vi "VIDoc Settings Editor.vi"(8 "Error in":errorcluster caption="Error in (no error)", 11 "VIDoc Settings Directory":path) -> (0 "Error out":errorcluster)   [LabVIEW 2023]
uses:
  Settings/VIDoc Settings/VIDoc Settings.lvclass
  Settings/Parser Settings/Parser Settings.lvclass
  Settings/Printer Settings/Printer Settings.lvclass
  <vilib>/event_ctls.llb/usereventprio.ctl
  VIDoc Editor/VIDocEditor.lvclass
  C:/Projects/Open Source/DMC VIDoc - Core/Source/Settings/VIDoc Settings/VIDoc Settings.lvclass
  C:/Projects/Open Source/DMC VIDoc - Core/Source/Editors/VIDoc Editor/VIDocEditor.lvclass
  C:/Projects/Open Source/DMC VIDoc - Core/Source/Settings/Parser Settings/Parser Settings.lvclass
  C:/Projects/Open Source/DMC VIDoc - Core/Source/Settings/Printer Settings/Printer Settings.lvclass
panel:
  in  "JSON Settings Path":path
  in  "Save":bool
  in  "Settings Sections":i32(listbox)
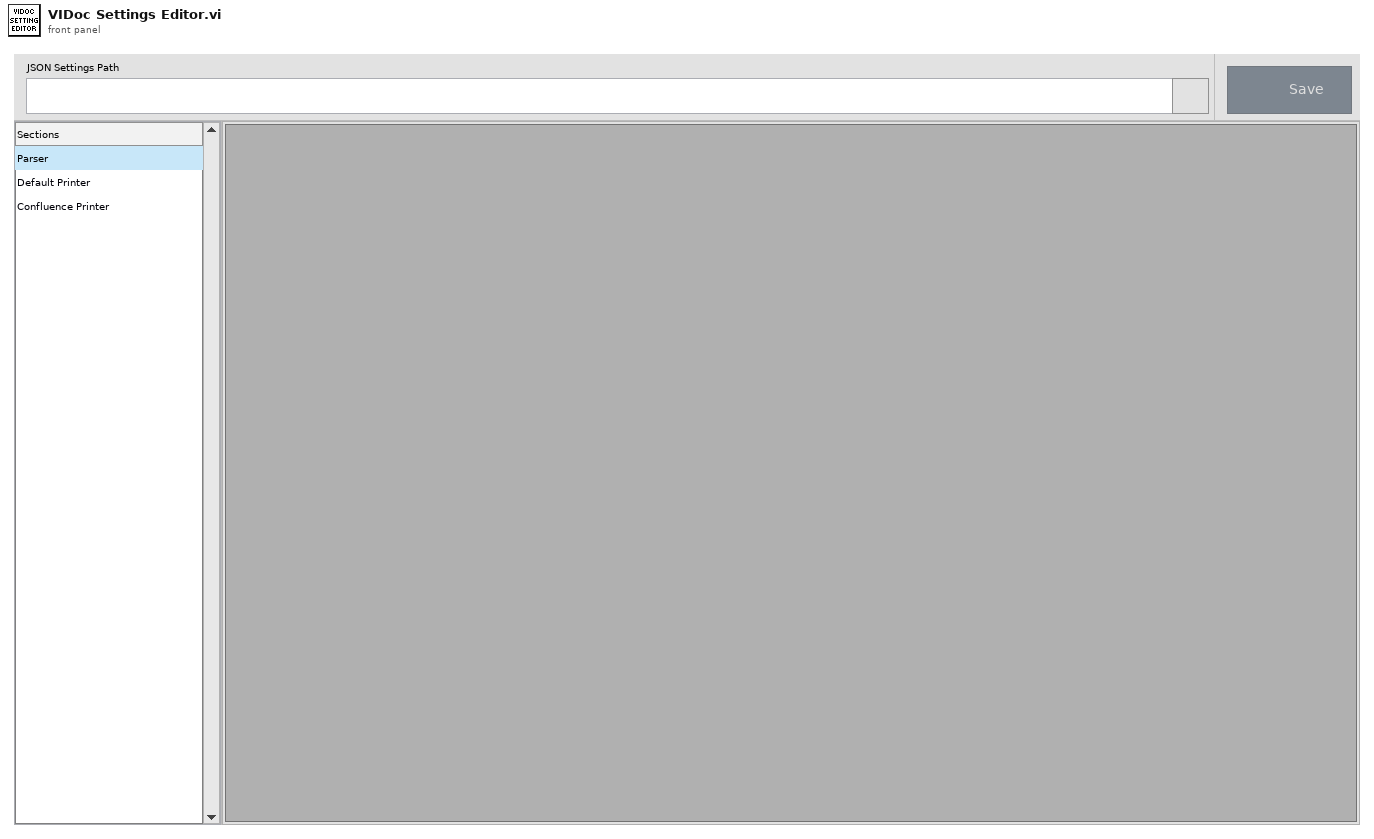
[diagram p1: front panel]
types:
  T1 = enum8{"Enabled", "Disabled", "Disabled and Grayed Out"}
  T2 = cluster{"JSON Settings Path":path, "Editors":refnum<class "VIDoc Settings.lvclass">[], "Current VI":refnum<vi>}
  T3 = typedef "VIDocEditor.lvclass/Editor Events Cluster.ctl" = cluster{"Close":refnum<user-event>, "Revert":refnum<user-event>, "Save":refnum<user-event>, "Changes?":refnum<user-event>}
  T4 = typedef "usereventprio.ctl" = enum32{"high priority", "normal priority"}
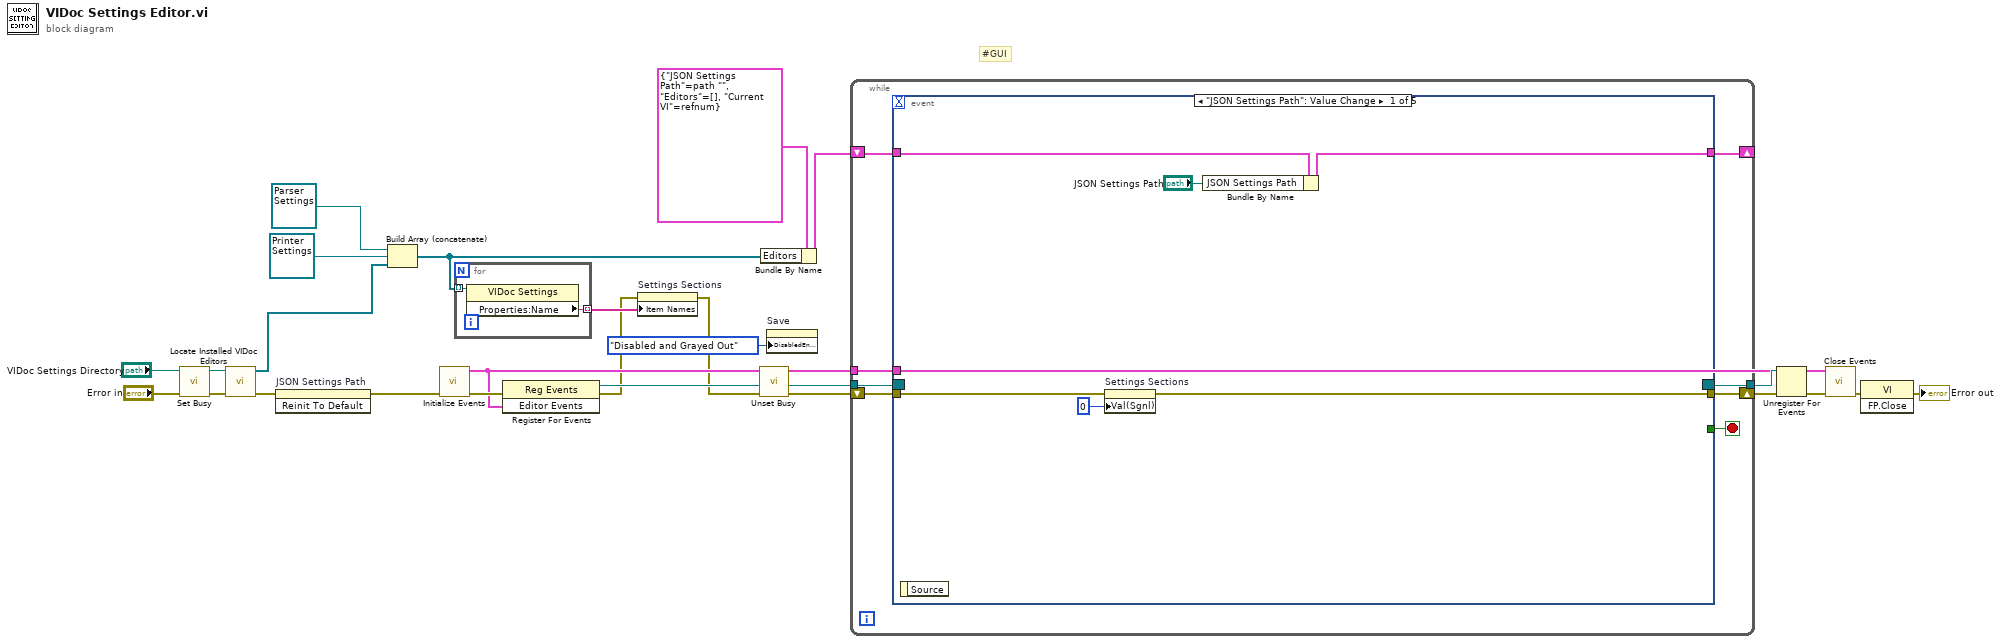
[diagram p0: block diagram]
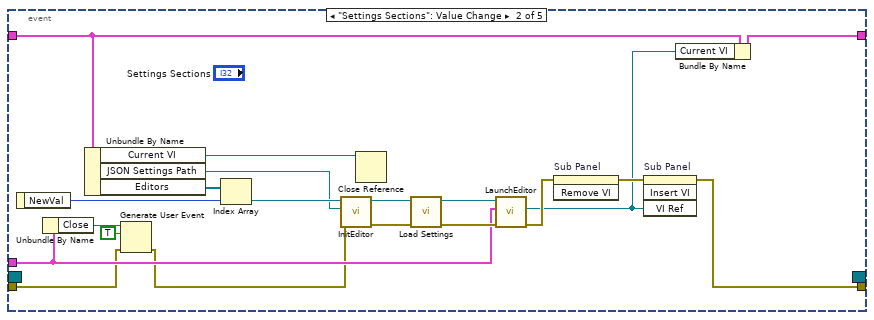
[diagram p2: hidden frame]
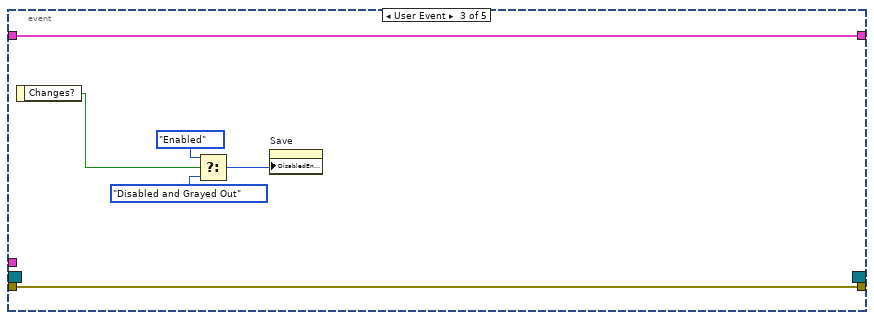
[diagram p3: hidden frame]
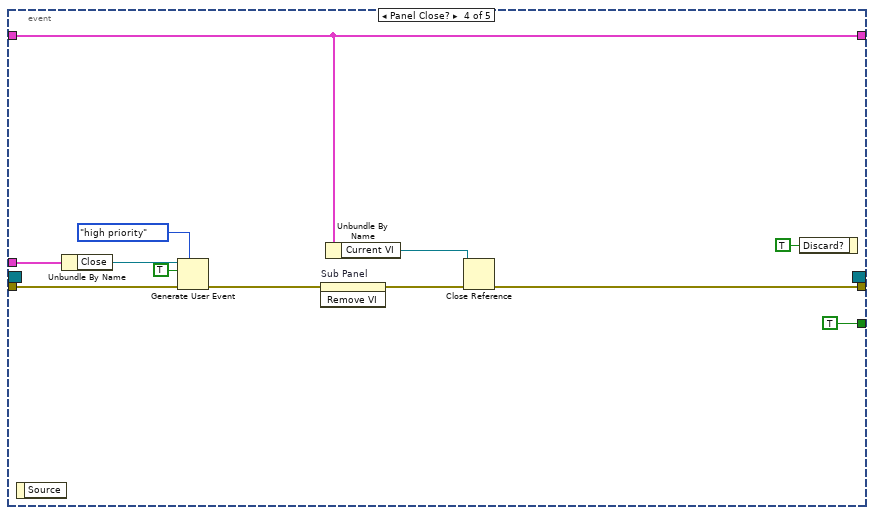
[diagram p4: hidden frame]
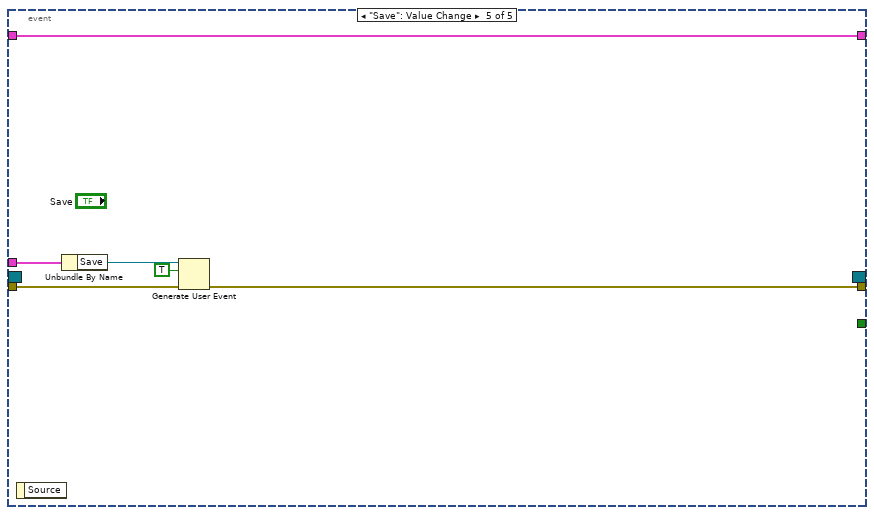
[diagram p5: hidden frame]
diagram:
  # "#GUI"
  n1 = call <vilib>:"Set Busy.vi"("error in (no error)"="Error in") -> ("error out"=w6:errorcluster)  [unwired: 9 in, 1 out]
  n2 = call "Locate Installed VIDoc Editors.vi"("Error in"=w6, "VIDoc Settings Directory"="VIDoc Settings Directory") -> ("Error out"=w12:errorcluster, "VIDoc Editors"=w11:refnum<class "VIDoc Settings.lvclass">[])  [unwired: 8 in]
  n3 = invoke on="JSON Settings Path" class="Path" method="Reinit To Default"(error in=w12) -> (error out=w14:errorcluster)  [unwired: 2 in, 2 out]
  n4 = Build Array (concatenate)(refnum<class "Parser Settings.lvclass"> refnum ("Parser Settings.lvclass"), refnum<class "Printer Settings.lvclass"> refnum ("Printer Settings.lvclass"), w11) -> (w8:refnum<class "VIDoc Settings.lvclass">[])
  n5 = call "Initialize Events.vi"("Error in"=w14) -> ("Error out"=w21:errorcluster, "Editor Events"=w16:T3)  [unwired: 9 in]
  n6 = for {
    tunnel: w8 -> [w26] mode=indexing
    tunnel: [w25] -> w9 mode=indexing
    n7 = property class="VIDoc Settings"(reference=w26) -> ("Properties:Name"=w25:string)  [unwired: 1 in, 2 out]
  }
  n8 = register-events(error in=w21, w16) -> (reference out=w20:refnum<event-registration>, error out=w5:errorcluster)  [unwired: 1 in]
  n9 = property on="Settings Sections" class="LstBox (strict)"(error in=w5, "Item Names"=w9) -> (error out=w4:errorcluster)  [unwired: 1 in, 1 out]
  n10 = call <vilib>:"Unset Busy.vi"("error in (no error)"=w4) -> ("error out"=w3:errorcluster)  [unwired: 10 in]
  n11 = Bundle By Name(cluster=T2 {"JSON Settings Path"=path "", "Editors"=[], "Current VI"=refnum} ("Cluster"), "Editors"=w8) -> (w23:T2)
  n12 = property on="Save" class="Bool"("DisabledEnum"=T1."Disabled and Grayed Out" ("Disabled")) -> ()  [unwired: 2 in, 2 out]
  n13 = while {
    shift-right: [w32] -> _
    shift-left: w23 -> [w34]
    shift-right: [w31] -> w19
    shift-left: w3 -> [w33]
    tunnel: w16 -> [w29]
    tunnel: w20 -> [w28]
    tunnel: [w27] -> w18
    stop <- w30 stop-if-true
    n14 = event shown="[0] \"JSON Settings Path\": Value Change" {
      selector: w28 -> [_ _ _ _ _]
      dyn-events: [_ _ _ _ _] -> w27
      timeout: _ -> [_ _ _ _ _]
      tunnel: w34 -> [w38 w60 w66 w69 w84]
      tunnel: w33 -> [w35 w41 w65 w77 w82]
      tunnel: [w40 w48 w66 w69 w84] -> w32
      tunnel: [w36 w53 w65 w70 w80] -> w31
      tunnel: [_ _ _ TRUE _] -> w30
      tunnel: w29 -> [_ w45 _ w75 w83]
      event "JSON Settings Path": Value Change {
        n15 = event-data() -> ()  [unwired: 1 in, 1 out]
        n16 = property on="Settings Sections" class="LstBox (strict)"(error in=w35, "Val(Sgnl)"=0 ("Value (Signaling)")) -> (error out=w36:errorcluster)  [unwired: 1 in, 1 out]
        n17 = Bundle By Name(cluster=w38, "JSON Settings Path"="JSON Settings Path") -> (w40:T2)
      }
      event "Settings Sections": Value Change {
        n18 = event-data() -> ("NewVal"=w58:i32)  [unwired: 1 in]
        n19 = Unbundle By Name(w45) -> ("Close"=w44:refnum<user-event>)
        n20 = Unbundle By Name(w60) -> ("Current VI"=w46:refnum<vi>, "JSON Settings Path"=w56:path, "Editors"=w59:refnum<class "VIDoc Settings.lvclass">[])
        n21 = Generate User Event(user event=w44, event data cluster=TRUE ("event data"), error in=w41) -> (error out=w42:errorcluster)  [unwired: 1 in, 1 out]
        n22 = Index Array(array=w59, index=w58) -> (element=w57:refnum<class "VIDoc Settings.lvclass">)
        n23 = call-dynamic "InitEditor.vi"("error in (no error)"=w42, "VIDoc Settings Path"=w56, "VIDoc Settings In"=w57) -> ("error out"=w51:errorcluster, "VIDoc Settings Out"=w52:refnum<class "VIDoc Settings.lvclass">)  [unwired: 7 in]
        n24 = Close Reference(reference=w46) -> ()  [unwired: 1 in, 1 out]
        n25 = call-dynamic "Load Settings.vi"("error in (no error)"=w51, "VIDoc Settings In"=w52) -> ("error out"=w49:errorcluster, "VIDoc Settings Out"=w50:refnum<class "VIDoc Settings.lvclass">)  [unwired: 8 in]
        n26 = call-dynamic "LaunchEditor.vi"("error in (no error)"=w49, "Editor Events"=w45, "VIDocEditor in"=w50) -> ("error out"=w54:errorcluster, "VI Refnum"=w47:refnum<vi>)  [unwired: 6 in, 1 out]
        n27 = invoke on="Sub Panel" class="SubPnl" method="Remove VI"(error in=w54) -> (error out=w55:errorcluster)  [unwired: 2 in, 2 out]
        n28 = invoke on="Sub Panel" class="SubPnl" method="Insert VI"(error in=w55, "VI Ref"=w47) -> (error out=w53:errorcluster)  [unwired: 2 in, 3 out]
        n29 = Bundle By Name(cluster=w60, "Current VI"=w47) -> (w48:T2)
      }
      event User Event {
        n30 = event-data() -> ("Changes?"=w63:bool)  [unwired: 1 in]
        n31 = Select(t=T1."Enabled", s=w63, f=T1."Disabled and Grayed Out" ("Disabled")) -> (s? t:f=w64:T1)
        n32 = property on="Save" class="Bool"("DisabledEnum"=w64) -> ()  [unwired: 2 in, 2 out]
      }
      event Panel Close? {
        n33 = event-data() -> ()  [unwired: 1 in, 1 out]
        n34 = Unbundle By Name(w75) -> ("Close"=w74:refnum<user-event>)
        n35 = Generate User Event(priority (normal)=usereventprio."high priority", user event=w74, event data cluster=TRUE ("event data"), error in=w77) -> (error out=w72:errorcluster)  [unwired: 1 out]
        n36 = invoke on="Sub Panel" class="SubPnl" method="Remove VI"(error in=w72) -> (error out=w71:errorcluster)  [unwired: 2 in, 2 out]
        n37 = Unbundle By Name(w69) -> ("Current VI"=w68:refnum<vi>)
        n38 = Close Reference(reference=w68, error in (no error)=w71) -> (error out=w70:errorcluster)
        n39 = event-data("Discard?"=TRUE) -> ()  [unwired: 1 in, 1 out]
      }
      event "Save": Value Change {
        n40 = event-data() -> ()  [unwired: 1 in, 1 out]
        n41 = Unbundle By Name(w83) -> ("Save"=w81:refnum<user-event>)
        n42 = Generate User Event(user event=w81, event data cluster=TRUE ("event data"), error in=w82) -> (error out=w80:errorcluster)  [unwired: 1 in, 1 out]
      }
    }
  }
  n43 = Unregister For Events(event registration refnum=w18, error in=w19) -> (error out=w17:errorcluster)
  n44 = call "Close Events.vi"("Error in"=w17, "Editor Events"=w16) -> ("Error out"=w2:errorcluster)  [unwired: 9 in]
  n45 = invoke class="VI" method="FP.Close"(error in=w2) -> (error out=→"Error out":errorcluster)  [unwired: 2 in, 2 out]
